vi "Test.vi"   [LabVIEW 2016]
doc: "This VI is called when test mode begins, and will automatically be terminated when it ends. You can add manual or automatic tests and invoke them from the dashboard."
uses:
  Global 4.vi
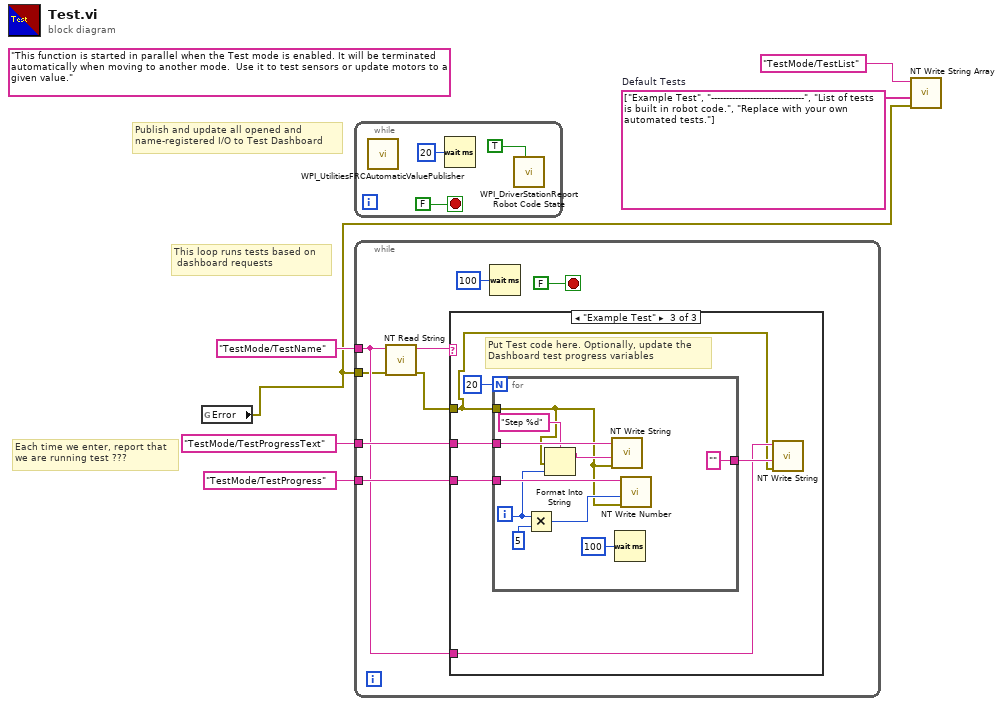
[diagram p0: block diagram]
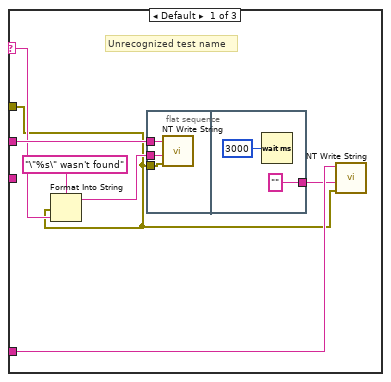
[diagram p2: hidden frame]
diagram:
  w3 = string[] ["Example Test", "-------------------------------", "List of tests is built in robot code.", "Replace with your own automated tests."]  # Default Tests
  (unwired) "This function is started in parallel when the Test mode is enabled. It will be terminated automatically when moving to another mode.  Use it to test sensors or update motors to a given value."
  # "This loop runs tests based on \n dashboard requests"
  # "Publish and update all opened and\nname-registered I/O to Test Dashboard"
  # "Each time we enter, report that\nwe are running test ???"
  n1 = global read "Global 4.vi" "Error"() -> (w1:errorcluster)
  n2 = while {
    stop <- FALSE stop-if-true
    n3 = call <vilib>:"WPI_UtilitiesFRCAutomaticValuePublisher.vi"() -> ()  [unwired: 12 in]
    n4 = Wait (ms)(milliseconds to wait=u32 20) -> ()  [unwired: 1 out]
    n5 = call <vilib>:"WPI_DriverStationReport Robot Code State.vi"("Test"=TRUE ("Autonomous")) -> ()  [unwired: 10 in, 1 out]
  }
  n6 = while {
    tunnel: "TestMode/TestName" ("Name") -> [w12]
    tunnel: "TestMode/TestProgressText" ("Name") -> [w15]
    tunnel: "TestMode/TestProgress" ("Name") -> [w14]
    tunnel: w1 -> [w10]
    stop <- FALSE stop-if-true
    n7 = call <vilib>:"NT Read String.vi"("error in"=w10, "Name"=w12) -> ("error out"=w11:errorcluster, "String"=w13:string)  [unwired: 8 in]
    n8 = case shown="\"Example Test\"" w13 {
      selector: w13 -> [w23 _ _]
      tunnel: w12 -> [w20 _ w31]
      tunnel: w15 -> [w24 _ w34]
      tunnel: w14 -> [_ _ w35]
      tunnel: w11 -> [w18 _ w30]
      frame Default {
        # "Unrecognized test name"
        n9 = Format Into String(format string="\"%s\" wasn't found" ("Name"), error in=w18, w23) -> (resulting string=w22:string)  [unwired: 1 in, 1 out]
        n10 = flat-sequence {
          tunnel: w24 -> [w26]
          tunnel: w22 -> [w27]
          tunnel: w18 -> [w25]
          tunnel: ["" ("Name")] -> w19
          frame #0 {
            n11 = call <vilib>:"NT Write String.vi"("error in"=w25, "String"=w27, "Name"=w26) -> ()  [unwired: 8 in, 1 out]
          }
          frame #1 {
            n12 = Wait (ms)(milliseconds to wait=u32 3000) -> ()  [unwired: 1 out]
          }
        }
        n13 = call <vilib>:"NT Write String.vi"("error in"=w18, "String"=w19, "Name"=w20) -> ()  [unwired: 8 in, 1 out]
      }
      frame "" {
        # "No test to run"
      }
      frame "Example Test" {
        # "Put Test code here. Optionally, update the\nDashboard test progress variables"
        n14 = for {
          N: 20 -> [_]
          tunnel: w35 -> [w45]
          tunnel: w34 -> [w43]
          tunnel: ["" ("String")] -> w32
          tunnel: w30 -> [w36]
          i -> [w40]
          n15 = Multiply(x=w40, y=u32 5 ("milliseconds to wait")) -> (x*y=w41:u32)
          n16 = Format Into String(format string="Step %d", error in=w36, w40) -> (resulting string=w38:string)  [unwired: 1 in, 1 out]
          n17 = call <vilib>:"NT Write String.vi"("error in"=w36, "String"=w38, "Name"=w43) -> ()  [unwired: 8 in, 1 out]
          n18 = Wait (ms)(milliseconds to wait=u32 100) -> ()  [unwired: 1 out]
          n19 = call <vilib>:"NT Write Number.vi"("error in"=w36, "Numeric"=w41, "Name"=w45) -> ()  [unwired: 8 in, 1 out]
        }
        n20 = call <vilib>:"NT Write String.vi"("error in"=w30, "String"=w32, "Name"=w31) -> ()  [unwired: 8 in, 1 out]
      }
    }
    n21 = Wait (ms)(milliseconds to wait=u32 100) -> ()  [unwired: 1 out]
  }
  n22 = call <vilib>:"NT Write String Array.vi"("error in"=w1, "String Array"=w3, "Name"="TestMode/TestList") -> ()  [unwired: 8 in, 1 out]
